vi "Test Steering Motion Profile.vi"(0 "Stop":bool) -> ()   [LabVIEW 2011]
panel:
  in  "KI":string
  in  "KD":string
  in  "KP":string
  in  "Steer Speed":string
  in  "Steer Deceleration":string
  in  "Steer Acceleration":string
  out "Galil Error":errorcluster
  in  "Initial Encoder Counts":string="0" caption="Enter number in encoder counts, 0 is middle, -650000 fully entended; 650000 fully retracted"
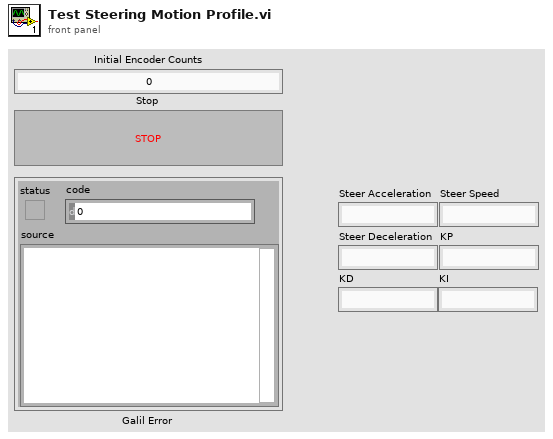
[diagram p1: front panel]
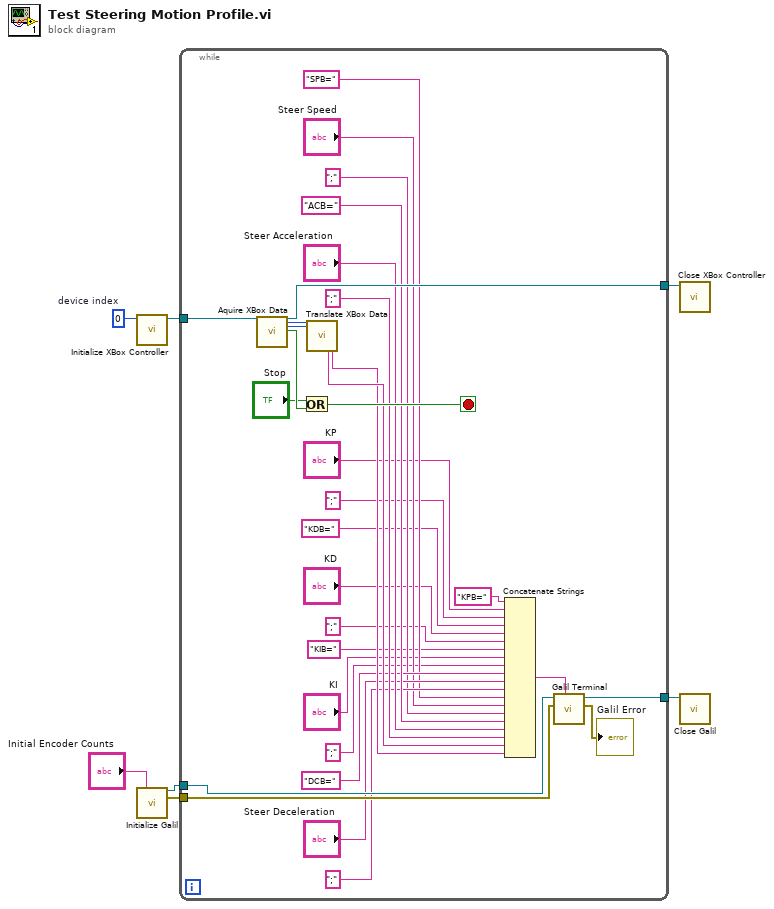
[diagram p0: block diagram]
diagram:
  w2 = 0  # device index
  n1 = call "Initialize XBox Controller.vi"("XBox Device Index"=w2) -> ("Device ID"=w6:refnum<k1>)  [unwired: 8 in, 2 out]
  n2 = call "Initialize Galil.vi"("Initial Encoder Counts"="Initial Encoder Counts") -> ("reference out 3"=w4:refnum<k7>, "error out 3"=w1:errorcluster)  [unwired: 9 in, 4 out]
  n3 = while {
    tunnel: [w39] -> w7
    tunnel: w6 -> [w38]
    tunnel: w4 -> [w33]
    tunnel: [w30] -> w3
    tunnel: w1 -> [w26]
    stop <- w35 stop-if-true
    n4 = call "Aquire XBox Data.vi"("device ID"=w38) -> ("device ID 2"=w39:refnum<k1>, "Steer Axis"=w37:i32, "Drive Axis"=w36:i32, "E-Stop (Button B)"=w34:bool)  [unwired: 21 in, 2 out]
    n5 = Or(x="Stop", y=w34) -> (x .or. y?=w35:bool)
    n6 = call "Translate XBox Data.vi"("Steer Axis"=w37, "Drive Axis"=w36) -> ("Steer Value Output String"=w28:string, "Drive Value Output String"=w27:string)  [unwired: 18 in, 6 out]
    n7 = Concatenate Strings("KPB=" ("string"), "KP", ";" ("string"), "KDB=" ("string"), "KD", ";" ("string"), "KIB=" ("string"), "KI", ";" ("string"), "DCB=" ("string"), "Steer Deceleration", ";" ("string"), "SPB=" ("string"), "Steer Speed", ";" ("string"), "ACB=" ("string"), "Steer Acceleration", ";" ("string"), w28, w27) -> (w32:string)
    n8 = call "Galil Terminal.vi"("Command Input"=w32, "Galil Error In"=w26, "reference out 2"=w33) -> ("Galil Error Out"=→"Galil Error":errorcluster, "reference out 3"=w30:refnum<k7>)  [unwired: 6 in, 1 out]
  }
  n9 = call "Close XBox Controller.vi"("Device ID In"=w7) -> ()  [unwired: 10 in, 1 out]
  n10 = call "Close Galil.vi"("reference out 2"=w3) -> ()  [unwired: 9 in, 2 out]
